vi "Get From Symbol Map Daemon.vi"(8 "error in (no error)":errorcluster, 10 "Symbol Name":string, 11 "TwinCAT ADS in":refnum<class "TwinCAT ADS.lvclass">) -> (0 "error out":errorcluster, 1 ".NET Symbol Information":refnum<k24>, 2 "Found?":bool, 3 "TwinCAT ADS out":refnum<class "TwinCAT ADS.lvclass">)   [LabVIEW 2018, in "TwinCAT ADS.lvclass"]
uses:
  TwinCAT ADS.lvclass
  TwinCAT.Ads
  TwinCAT ADS.lvclass/TwinCAT ADS.ctl
  Controls/Daemon Message.ctl
  Get Symbol Map.vi
  Format String.vi
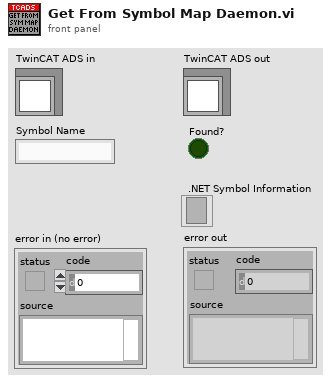
[diagram p1: front panel]
types:
  T1 = typedef "TwinCAT ADS.lvclass/Daemon Message.ctl" = cluster{"Symbol Name":string, "Occurrence":refnum<k4>}
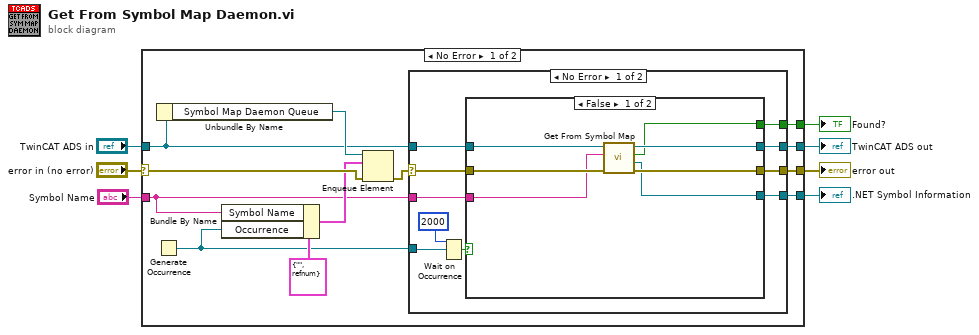
[diagram p0: block diagram]
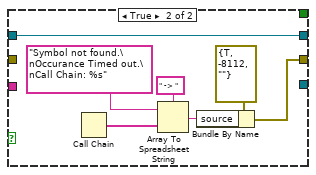
[diagram p2: hidden frame]
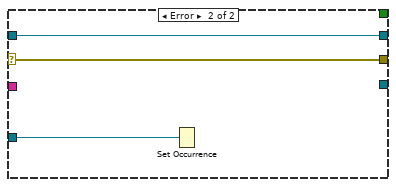
[diagram p3: hidden frame]
diagram:
  n1 = case shown="No Error" "error in (no error)" {
    selector: "error in (no error)" -> [w18 w47]
    tunnel: "TwinCAT ADS in" -> [w13 w48]
    tunnel: "Symbol Name" -> [w12 _]
    tunnel: [w10 w47] -> w5
    tunnel: [w11 w48] -> w4
    tunnel: [w9 _] -> w2
    tunnel: [w8 _] -> w1
    frame No Error {
      n2 = Generate Occurrence() -> (w14:refnum<k4>)
      n3 = Unbundle By Name(w13) -> ("Symbol Map Daemon Queue"=w19:refnum<queue>)
      n4 = Bundle By Name(cluster=T1 {"Symbol Name"="", "Occurrence"=refnum} ("Daemon Message"), "Symbol Name"=w12, "Occurrence"=w14) -> (w16:T1)
      n5 = Enqueue Element(queue=w19, element=w16, error in (no error)=w18) -> (error out=w15:errorcluster)  [unwired: 1 in, 2 out]
      n6 = case shown="No Error" w15 {
        selector: w15 -> [w25 w45]
        tunnel: w14 -> [w29 w46]
        tunnel: w13 -> [w26 w44]
        tunnel: w12 -> [w24 _]
        tunnel: [w23 w44] -> w11
        tunnel: [w22 w45] -> w10
        tunnel: [w21 _] -> w9
        tunnel: [w20 _] -> w8
        frame No Error {
          n7 = Wait on Occurrence(2:w29, 3:2000 ("ms timeout (-1)")) -> (0:w27:bool)  [unwired: 1 in]
          n8 = case shown="False" w27 {
            tunnel: w26 -> [w36 w43]
            tunnel: w25 -> [w35 _]
            tunnel: w24 -> [w34 _]
            tunnel: [w33 w43] -> w23
            tunnel: [w32 w37] -> w22
            tunnel: [w31 _] -> w21
            tunnel: [w30 _] -> w20
            frame False {
              n9 = call "Get From Symbol Map.vi"("error in (no error)"=w35, "Symbol Name"=w34, "TwinCAT ADS in"=w36) -> ("error out"=w32:errorcluster, ".NET Symbol Information"=w31:refnum<k24>, "Found?"=w30:bool, "TwinCAT ADS out"=w33:refnum<class "TwinCAT ADS.lvclass">)  [unwired: 5 in]
            }
            frame True {
              n10 = Call Chain() -> (call chain=w42:string[])
              n11 = Array To Spreadsheet String(delimiter (Tab)=" -> ", array=w42, 3:"Symbol not found.\nOccurance Timed out.\nCall Chain: %s" ("format string")) -> (spreadsheet string=w38:string)
              n12 = Bundle By Name(cluster=errorcluster {"status"=TRUE, "code"=-8112, "source"=""} ("error out"), "source"=w38) -> (w37:errorcluster)
            }
          }
        }
        frame Error {
          n13 = Set Occurrence(w46) -> ()
        }
      }
    }
    frame Error {
    }
  }
  "error out" <- w5
  "TwinCAT ADS out" <- w4
  ".NET Symbol Information" <- w2
  "Found?" <- w1
